vi "웹서버 수정 버전 2.vi"(5 "불리언 센서 정지":bool, 7 "온도센서 정지":bool, 8 "참조 번호 입력":T1 caption="client handle out", 9 "lines":tag caption="라인", 10 "physical channels":tag caption="물리적 채널", 11 "thermocouple type":i32(ring)=10072 caption="열전쌍 타입" items=["J"=10072, "K"=10073, "N"=10077, "R"=10082, "S"=10085, "T"=10086, "B"=10047, "E"=10055]) -> (0 "F포맷 문자열":string[](array[string]), 1 "참조 번호 출력 2":T1 caption="client handle out", 2 "불리언값":string, 3 "온도값":string)   [LabVIEW 2019]
uses:
  <vilib>/httpClient/ClientHandle.ctl
  <vilib>/httpClient/LabVIEWHTTPClient.lvlib
panel:
  out "data":bool[](array[boolean]) caption="데이터"
  out "headers 4":string caption="연결확인 메세지 출력"
  out "10진수 문자열":string[](array[string])
  out "숫자형":i32
  out "headers 3":string caption="연결확인 메세지 출력"
  out "참조 번호 출력":T1 caption="client handle out"
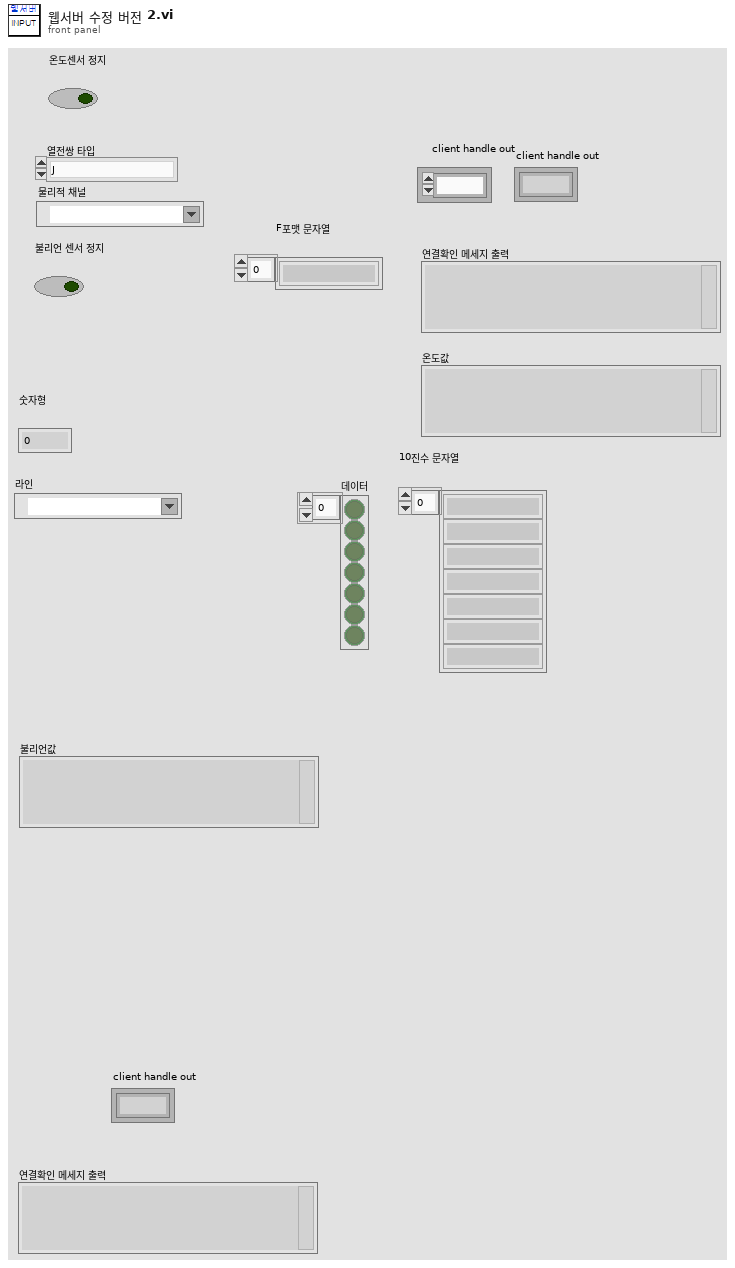
[diagram p1: front panel]
types:
  T1 = typedef "LabVIEWHTTPClient.lvlib/ClientHandle.ctl" = refnum<k1>
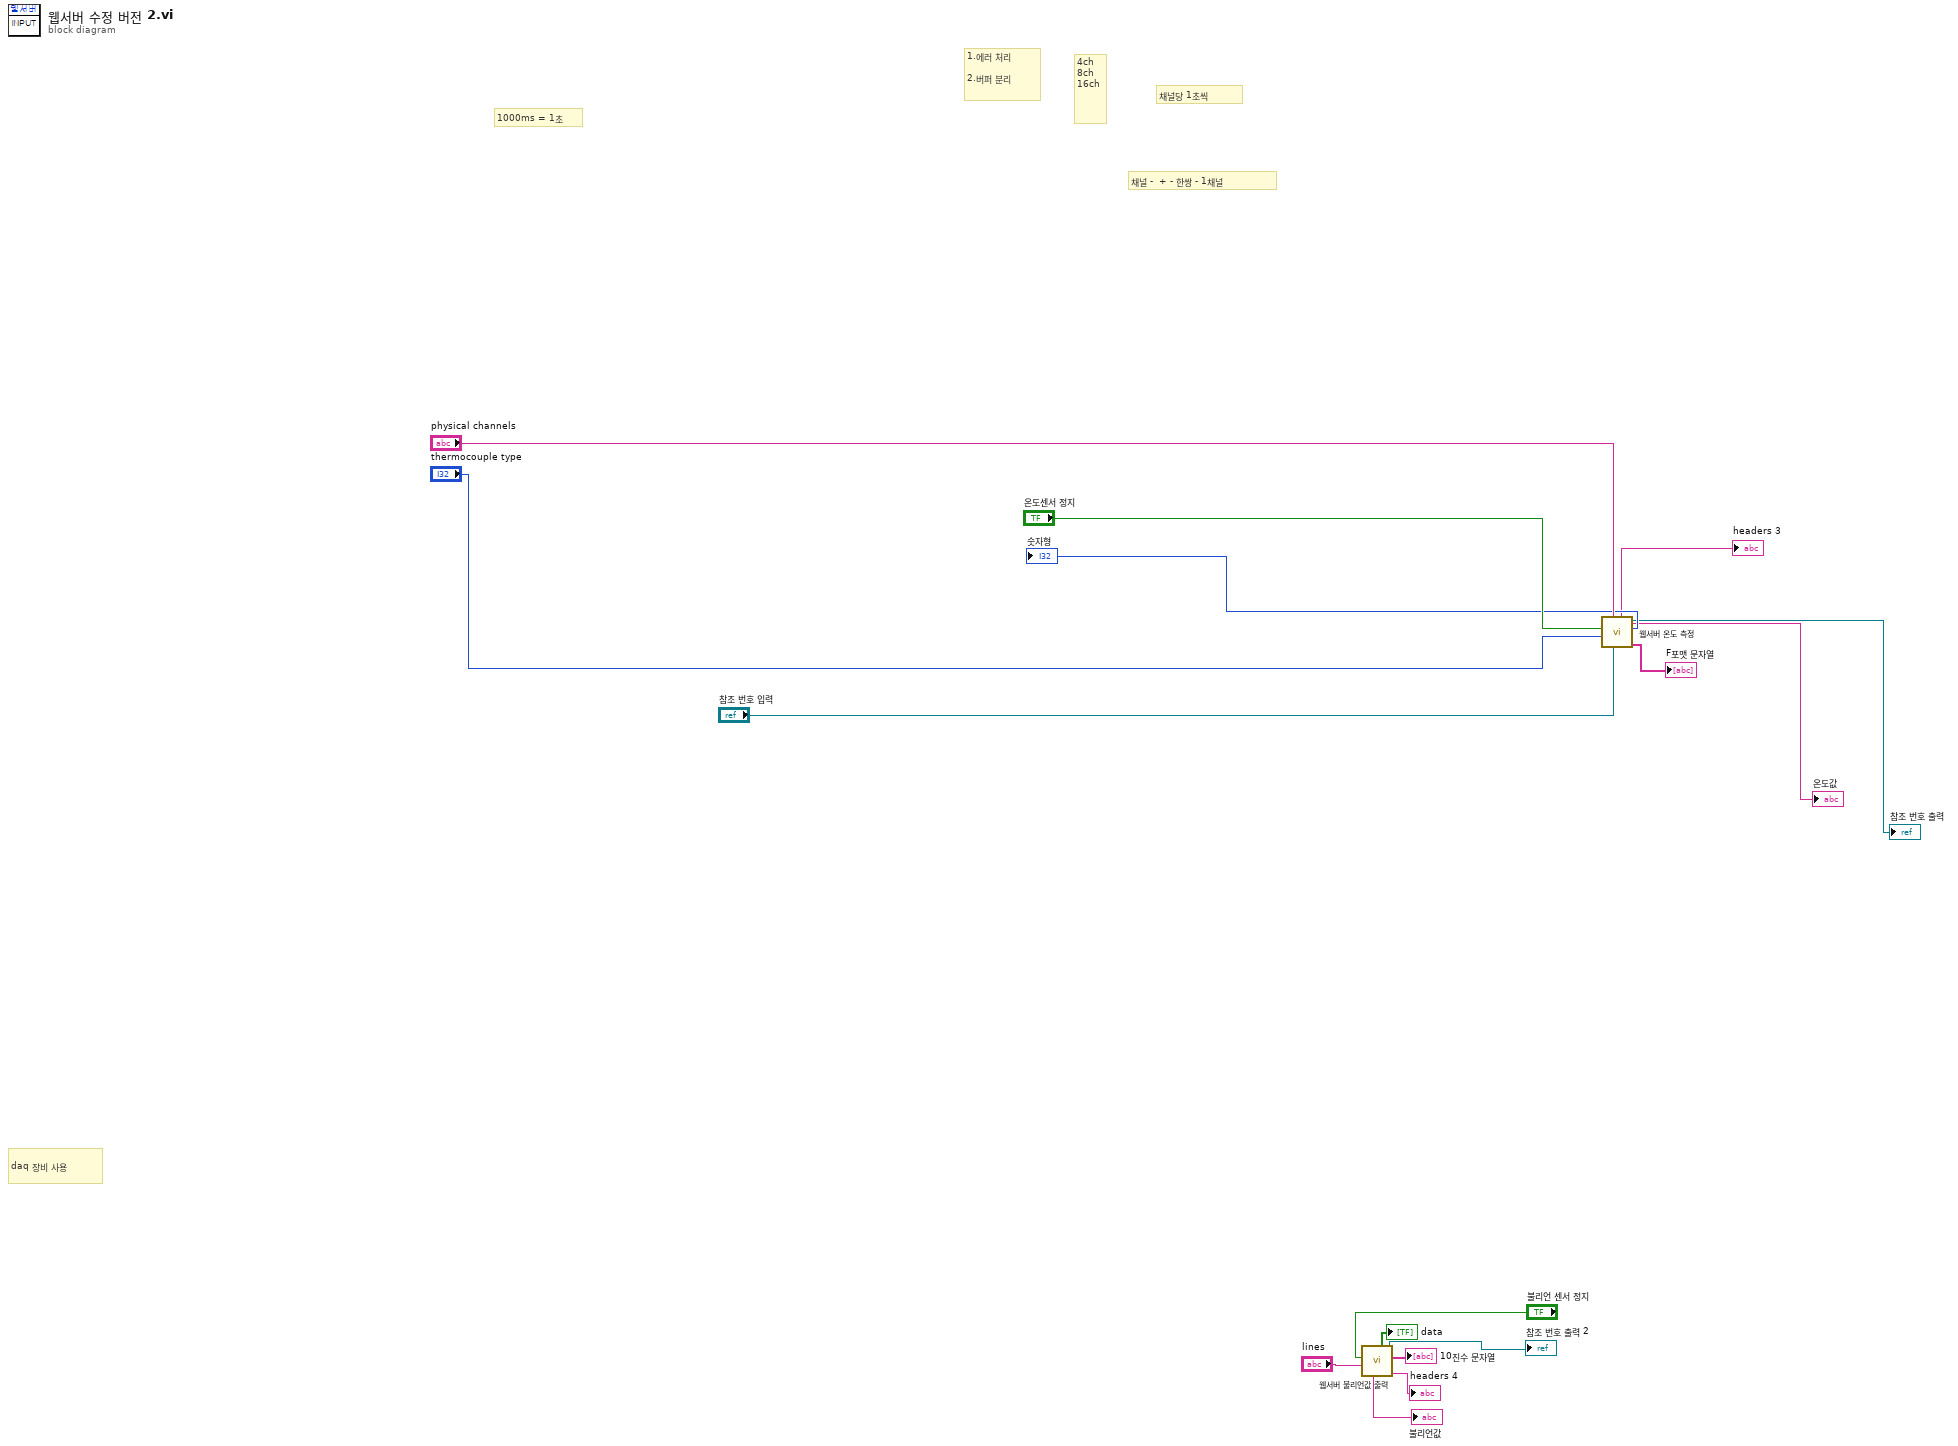
[diagram p0: block diagram]
diagram:
  # "1000ms = 1초"
  # "daq 장비 사용"
  # "1.에러 처리 \n\n2.버퍼 분리"
  # "채널 -  + - 한쌍 - 1채널"
  # "채널당 1초씩"
  # "4ch\n8ch\n16ch"
  n1 = call "웹서버 불리언값 출력.vi"("lines"="lines", "불리언 센서 정지"="불리언 센서 정지") -> ("headers 4"=→"headers 4":string, "10진수 문자열"=→"10진수 문자열":string[], "참조 번호 출력"=→"참조 번호 출력 2":T1, "data"=→"data":bool[], "불리언값"=→"불리언값":string)  [unwired: 3 in, 2 out]
  n2 = call "웹서버 온도 측정.vi"("참조 번호 입력"="참조 번호 입력", "physical channels"="physical channels", "thermocouple type"="thermocouple type", "온도센서 정지"="온도센서 정지") -> ("F포맷 문자열"=→"F포맷 문자열":string[], "숫자형"=→"숫자형":i32, "참조 번호 출력"=→"참조 번호 출력":T1, "headers 3"=→"headers 3":string, "온도값"=→"온도값":string)  [unwired: 2 in, 1 out]
